vi "F Dwf Analog Impedance Probe Get.vi"(8 "error in (no error)":errorcluster, 9 "pfaradCap":dbl, 10 "pohmRes":dbl, 11 "hdwf":i32) -> (0 "error out":errorcluster, 1 "pfaradCap out":dbl, 2 "pohmRes out":dbl, 3 "function return":i32)   [LabVIEW 2021, in "Olasdwf.lvlib"]
doc: "DWFAPI int FDwfAnalogImpedanceProbeGet(HDWF hdwf, double *pohmRes, double *pfaradCap);"
uses:
  Olasdwf.lvlib
  Windows/System32/dwf.dll
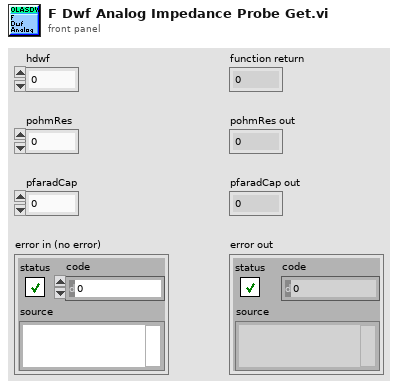
[diagram p1: front panel]
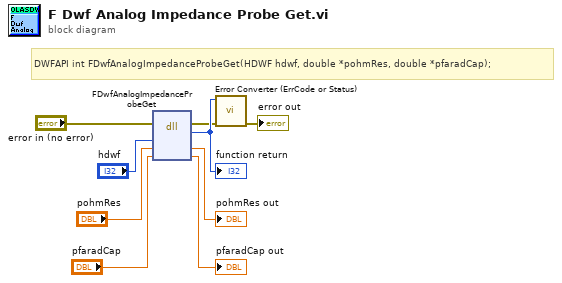
[diagram p0: block diagram]
diagram:
  # "DWFAPI int FDwfAnalogImpedanceProbeGet(HDWF hdwf, double *pohmRes, double *pfaradCap);"
  n1 = dll-call lib="/Windows/System32/dwf.*" fn="FDwfAnalogImpedanceProbeGet"(error in="error in (no error)", "hdwf"="hdwf", "pohmRes"="pohmRes", "pfaradCap"="pfaradCap") -> (error out=w2:errorcluster, w9:i32, "pohmRes"=→"pohmRes out":dbl, "pfaradCap"=→"pfaradCap out":dbl)  [unwired: 3 in, 1 out]
  "function return" <- w9
  n2 = call "Error Converter (ErrCode or Status).vi"("error in (no error)"=w2, "error code"=w9) -> ("error out"=→"error out":errorcluster)  [unwired: 9 in]
